vi "CreateDatabase.vi"() -> ()   [LabVIEW 2021, in "XNET-CAN-Signal-Logger.lvlib"]
uses:
  <vilib>/xnet/xnet.llb/XNET Database Create (Cluster).vi
  <vilib>/xnet/xnet.llb/XNET Database Create (Frame).vi
  <vilib>/xnet/xnet.llb/XNET Database Create (Signal).vi
  XNET-CAN-Signal-Logger.lvlib
  <resource>/objmgr/xnet.rc
panel:
  out "Num Signals":i32
  out "error out":errorcluster
  in  "filepath (empty)":path=path "C:/Users/NI/Desktop/NIO DongZulong FlexLogger XNET/ManyXnetChannels.xml"
  in  "Num Frames":i32=128
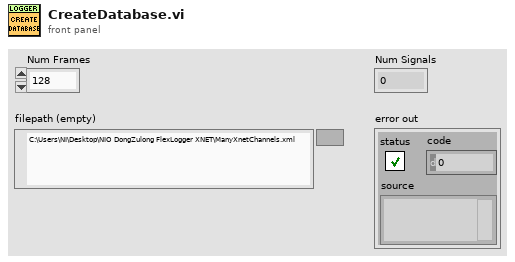
[diagram p1: front panel]
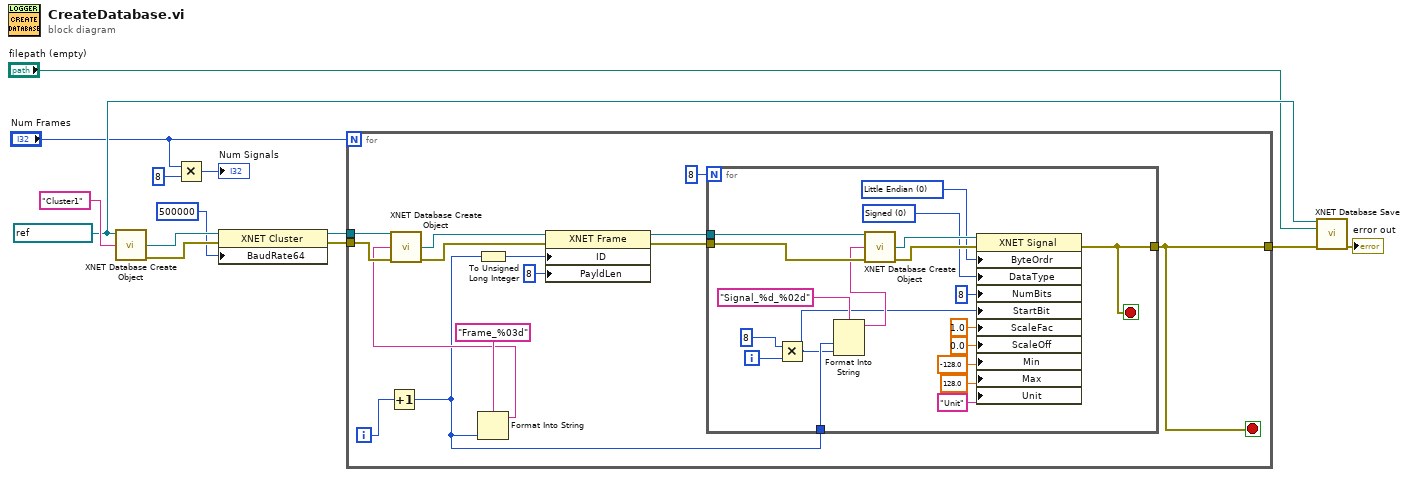
[diagram p0: block diagram]
diagram:
  w7 = refnum<k21> ":memory:" ("XNET Database")
  n1 = call-poly <vilib>:"XNET Database Create Object.vi"("database in"=w7, "cluster name"="Cluster1") -> ("cluster out"=w11:refnum<k21>, "error out"=w12:errorcluster)  [unwired: 11 in, 1 out]
  n2 = Multiply(x="Num Frames", y=8) -> (x*y=→"Num Signals":i32)
  n3 = property class="XNET Cluster"(reference=w11, error in=w12, "BaudRate64"=u64 500000 ("64bit Baud Rate")) -> (reference out=w9:refnum<k21>, error out=w8:errorcluster)
  n4 = for {
    N: "Num Frames" -> [_]
    tunnel: w9 -> [w27]
    tunnel: w8 -> [w26]
    tunnel: [w15] -> w6
    i -> [w23]
    stop <- w15 stop-if-true
    n5 = Increment(x=w23) -> (x+1=w14:i32)
    n6 = To Unsigned Long Integer(number=w14) -> (unsigned 32bit integer=w18:u32)
    n7 = Format Into String(format string="Frame_%03d", w14) -> (resulting string=w19:string)  [unwired: 2 in, 1 out]
    n8 = call-poly <vilib>:"XNET Database Create Object.vi"("cluster in"=w27, "frame name"=w19, "error in (no error)"=w26) -> ("frame out"=w25:refnum<k21>, "error out"=w24:errorcluster)  [unwired: 10 in, 1 out]
    n9 = property class="XNET Frame"(reference=w25, error in=w24, "ID"=w18, "PayldLen"=u32 8 ("Payload Length")) -> (reference out=w20:refnum<k21>, error out=w16:errorcluster)
    n10 = for {
      N: 8 -> [_]
      tunnel: w20 -> [w46]
      tunnel: w16 -> [w45]
      tunnel: [w37] -> w15
      tunnel: w14 -> [w34]
      i -> [w39]
      stop <- w37 stop-if-true
      w41 = u32 0 items=["Signed", "Unsigned", "IEEE Float", "Byte Array"] ("Data Type")
      w42 = u32 0 items=["Little Endian", "Big Endian"] ("Byte Order")
      n11 = Multiply(x=8 ("y"), y=w39) -> (x*y=w29:i32)
      n12 = Format Into String(format string="Signal_%d_%02d", w34, w29) -> (resulting string=w32:string)  [unwired: 2 in, 1 out]
      n13 = call-poly <vilib>:"XNET Database Create Object.vi"("frame in"=w46, "signal name"=w32, "error in (no error)"=w45) -> ("signal out"=w44:refnum<k21>, "error out"=w43:errorcluster)  [unwired: 10 in, 1 out]
      n14 = property class="XNET Signal"(reference=w44, error in=w43, "ByteOrdr"=w42, "DataType"=w41, "NumBits"=u32 8 ("Number of Bits"), "StartBit"=w29, "ScaleFac"=1.0 ("Scaling Factor"), "ScaleOff"=0.0 ("Scaling Offset"), "Min"=-128.0 ("Minimum Value"), "Max"=128.0 ("Maximum Value"), "Unit"="Unit") -> (error out=w37:errorcluster)  [unwired: 1 out]
    }
  }
  n15 = call <vilib>:"XNET Database Save.vi"("database in"=w7, "filepath (empty)"="filepath (empty)", "error in (no error)"=w6) -> ("error out"=→"error out":errorcluster)  [unwired: 11 in, 1 out]
